vi "Find LabView Version.vi"(4 "Lv version":refnum<vi>, 5 "LabView Version File":path=path "C:/Weekly Runs/Weekly_runs_General/Select_verison.txt") -> (0 "error out":errorcluster)   [LabVIEW 2015]
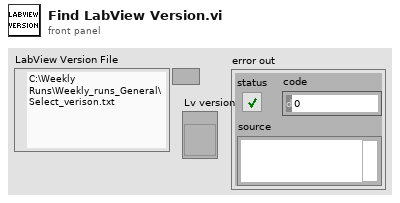
[diagram p1: front panel]
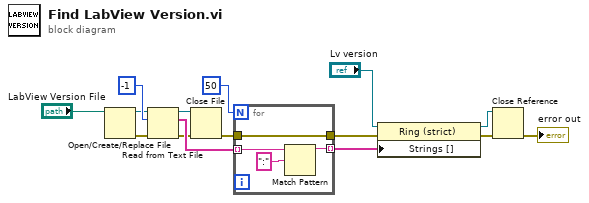
[diagram p0: block diagram]
diagram:
  n1 = Open/Create/Replace File(file path (use dialog)="LabView Version File") -> (refnum out=w4:refnum<file>, error out=w5:errorcluster)  [unwired: 5 in, 1 out]
  n2 = Read from Text File(file (use dialog)=w4, count=-1, error in=w5) -> (refnum out=w15:refnum<file>, text=w13:string[], error out=w10:errorcluster)  [unwired: 1 in, 1 out]
  n3 = Close File(refnum=w15, error in=w10) -> (error out=w11:errorcluster)  [unwired: 1 out]
  n4 = for {
    N: 50 -> [_]
    tunnel: [w19] -> w6 mode=indexing
    tunnel: [w18] -> w9
    tunnel: w11 -> [w18]
    tunnel: w13 -> [w16] mode=indexing
    n5 = Match Pattern(string=w16, regular expression=":") -> (before substring=w19:string)  [unwired: 1 in, 3 out]
  }
  n6 = property class="Ring (strict)"(reference="Lv version", error in=w9, "Strings []"=w6) -> (reference out=w7:refnum<vi>, error out=w8:errorcluster)
  n7 = Close Reference(reference=w7, error in (no error)=w8) -> (error out=→"error out":errorcluster)
